vi "color.vi"(4 "数组":dbl[][](array[numeric]), 5 "数组 3":dbl[][](array[numeric]), 6 "数组 2":dbl[][](array[numeric]), 7 "New Image 3":T1, 9 "New Image 2":T1, 10 "New Image":T1, 11 "引用句柄输入":T1) -> (3 "引用句柄输出":T1(plugin-control))   [LabVIEW 2018]
uses:
  <vilib>/vision/Image Controls.llb/IMAQ Image.ctl
  <vilib>/vision/NI_Vision_Development_Module.lvlib
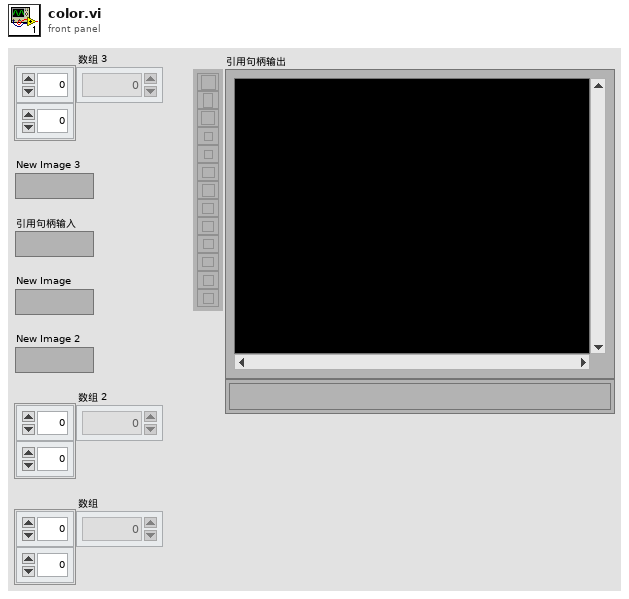
[diagram p1: front panel]
types:
  T1 = typedef "IMAQ Image.ctl" = refnum<image>
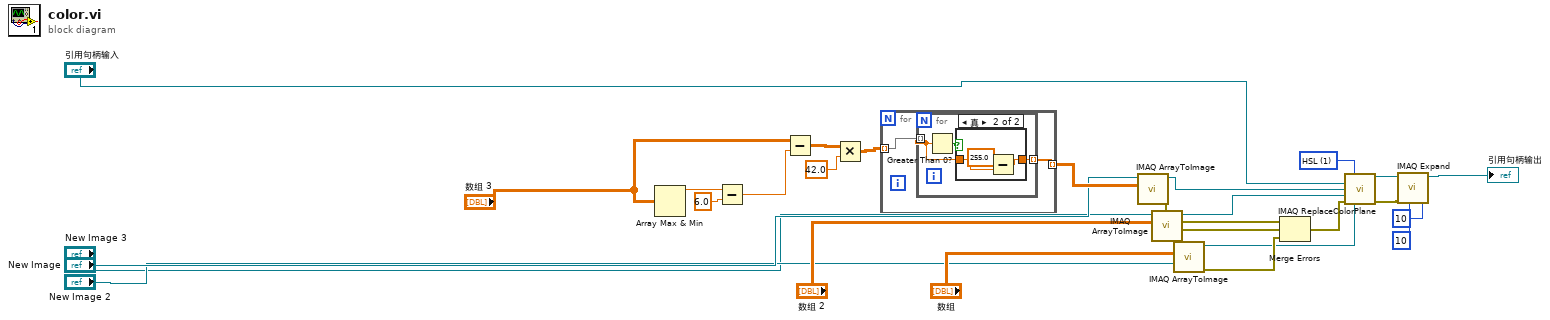
[diagram p0: block diagram]
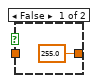
[diagram p2: hidden frame]
diagram:
  w9 = u16 1 items=["RGB", "HSL", "HSV", "HSI"] ("Color Mode")
  n1 = Array Max & Min(array="数组 3") -> (max value=w25:dbl)  [unwired: 3 out]
  n2 = Subtract(x=w25, y=6.0) -> (x-y=w24:dbl)
  n3 = Subtract(x="数组 3", y=w24) -> (x-y=w26:dbl[][])
  n4 = Multiply(x=w26, y=42.0) -> (x*y=w8:dbl[][])
  n5 = for {
    tunnel: w8 -> [w29] mode=indexing
    tunnel: [w28] -> w22 mode=indexing
    n6 = for {
      tunnel: w29 -> [w31] mode=indexing
      tunnel: [w30] -> w28 mode=indexing
      n7 = Greater Than 0?(x=w31) -> (x > 0?=w32:bool)
      n8 = case shown="真" w32 {
        tunnel: w31 -> [_ w35]
        tunnel: [255.0 w34] -> w30
        frame False {
        }
        frame True {
          n9 = Subtract(x=255.0, y=w35) -> (x-y=w34:dbl)
        }
      }
    }
  }
  n10 = call "IMAQ ArrayToImage"("Image Pixels (U8)"=w22, "Image"="New Image") -> ("error out"=w18:errorcluster, "Image Out"=w13:T1)  [unwired: 8 in]
  n11 = call "IMAQ ArrayToImage"("Image Pixels (U8)"="数组 2", "Image"="New Image 3") -> ("error out"=w19:errorcluster, "Image Out"=w14:T1)  [unwired: 8 in]
  n12 = call "IMAQ ArrayToImage"("Image Pixels (U8)"="数组", "Image"="New Image 2") -> ("error out"=w20:errorcluster, "Image Out"=w15:T1)  [unwired: 8 in]
  n13 = Merge Errors(w18, w19, w20) -> (w21:errorcluster)
  n14 = call "IMAQ ReplaceColorPlane"("Color Mode"=w9, "Image Dst"="引用句柄输入", "Red or Hue Plane"=w13, "Green or Sat Plane"=w14, "error in (no error)"=w21, "Blue or Luma or Val or Inten Plane"=w15) -> ("Image Dst Out"=w12:T1, "error out"=w17:errorcluster)  [unwired: 8 in]
  n15 = call "IMAQ Expand"("Y Duplication Step"=10, "error in (no error)"=w17, "X Duplication Step"=10, "Image Src"=w12) -> ("Image Dst Out"=→"引用句柄输出":T1)  [unwired: 6 in, 1 out]
